vi "Display - Update_SubVI.vi"(4 "Error Msg In":string, 5 "Lat":dbl, 6 "Enum":T1, 7 "GPS Connected?":bool, 8 "error in (no error)":errorcluster, 9 "Heart Rate":dbl, 10 "Distance Run":dbl, 11 "Time Elapsed":dbl) -> (0 "error out":errorcluster)   [LabVIEW 2021]
uses:
  Main - States_SubVI.ctl
  <vilib>/myRIO/Instrument Drivers/Onboard IO/I2C/typedefs/I2C User Configuration.ctl
  <vilib>/myRIO/Instrument Drivers/Onboard IO/I2C/typedefs/I2C Transfer Rate.ctl
  <vilib>/myRIO/Instrument Drivers/Onboard IO/I2C/typedefs/I2C Reference.ctl
  <vilib>/myRIO/Common/Instrument Driver Framework/Utilities/typedefs/myRIO Generic Hardware Reference.ctl
  <vilib>/myRIO/Common/Instrument Driver Framework/Utilities/typedefs/Hardware Version Enum.ctl
  <vilib>/myRIO/Common/Instrument Driver Framework/Utilities/typedefs/myRIO v1.0 Reference.ctl
  <vilib>/myRIO/Common/Instrument Driver Framework/Utilities/typedefs/Generic FPGA Reference.ctl
  <vilib>/myRIO/Common/Instrument Driver Framework/myRIO v1.0/I2C/typedefs/I2C Channels Enum.ctl
  <vilib>/myRIO/Instrument Drivers/Onboard IO/I2C/typedefs/I2C Configuration.ctl
  <vilib>/userDefined/High Color/nirio_resource_hc.ctl
  <vilib>/myRIO/Common/Instrument Driver Framework/Utilities/vis/Is FPGA Ref Available.vi
  <vilib>/myRIO/Common/Instrument Driver Framework/myRIO v1.0/I2C/vis/myRIO v1.1 Open I2C.vi
  <vilib>/myRIO/Instrument Drivers/Onboard IO/I2C/vis/Configure.vi
  <vilib>/myRIO/Instrument Drivers/Onboard IO/I2C/vis/Write.vi
  <vilib>/myRIO/Common/Instrument Driver Framework/Utilities/vis/Validate Channels.vi
  <vilib>/myRIO/Common/Instrument Driver Framework/myRIO v1.0/I2C/vis/myRIO v1.0 Reserve I2C.vi
  <vilib>/myRIO/Common/Instrument Driver Framework/myRIO v1.0/I2C/vis/myRIO v1.0 Build MUX Configuration I2C.vi
  <vilib>/myRIO/Common/Instrument Driver Framework/myRIO v1.0/Resource Manager/vis/myRIO v1.0 Reserve Channel List.vi
  <vilib>/myRIO/Common/Instrument Driver Framework/myRIO v1.0/Resource Manager/vis/myRIO v1.0 Create Configuration List.vi
  <vilib>/myRIO/Common/Instrument Driver Framework/myRIO v1.0/Resource Manager/vis/myRIO v1.0 Reserve Channel.vi
  <vilib>/myRIO/Common/Instrument Driver Framework/myRIO v1.0/Resource Manager/vis/myRIO v1.0 Unreserve Channel.vi
  <vilib>/myRIO/Common/Instrument Driver Framework/myRIO v1.0/Resource Manager/vis/myRIO v1.0 Build Mutex Name.vi
  <vilib>/Utility/VariantDataType/GetNumericInfo.vi
  <vilib>/Utility/error.llb/Error Cluster From Error Code.vi
  <vilib>/myRIO/Common/Instrument Driver Framework/myRIO v1.0/myRIO v1.1 Open.vi
  <vilib>/myRIO/Common/Instrument Driver Framework/Utilities/vis/IO Manager.vi
  <vilib>/myRIO/Common/Instrument Driver Framework/Utilities/vis/Configuration Manager.vi
  <vilib>/myRIO/Common/Instrument Driver Framework/myRIO v1.0/Resource Manager/vis/myRIO v1.0 Configure IO.vi
  <vilib>/myRIO/Common/Instrument Driver Framework/myRIO v1.0/myRIO v1.0 Close.vi
  <vilib>/myRIO/Common/Instrument Driver Framework/myRIO v1.0/I2C/vis/myRIO v1.0 Configure I2C.vi
  <vilib>/myRIO/Common/Instrument Driver Framework/myRIO v1.0/I2C/vis/myRIO v1.0 Write I2C.vi
  <vilib>/myRIO/Express VI/Onboard IO/I2C/I2C Express VI.xnode
  <vilib>/myRIO/Instrument Drivers/Onboard IO/I2C/vis/myRIO I2C Open.xnode
  <vilib>/myRIO/Instrument Drivers/Onboard IO/I2C/I2C.lvlib
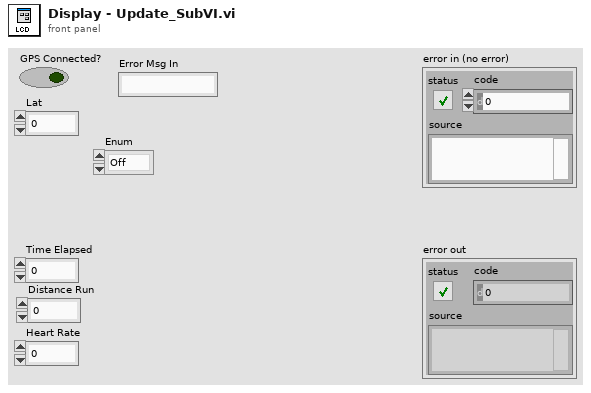
[diagram p1: front panel]
types:
  T1 = typedef "Main - States_SubVI.ctl" = enum16{"Off", "Record", "Upload", "Shutdown", "Error"}
  T2 = typedef "I2C.lvlib/I2C Reference.ctl" = cluster{"myRIO Reference":T3, "I2C Channels Enum":T7, "I2C Configuration":T8}
  T3 = typedef "myRIO Generic Hardware Reference.ctl" = cluster{"myRIO Model":T4, "myRIO Hardware Reference":T5}
  T4 = typedef "Hardware Version Enum.ctl" = enum16{"Unknown", "myRIO-1900", "myRIO-1950", "roboRIO", "NI ELVIS RIO CM", "ELVIS III"}
  T5 = typedef "myRIO v1.0 Reference.ctl" = cluster{"Generic FPGA Reference":T6, "Allow multiple opens":bool}
  T6 = typedef "Generic FPGA Reference.ctl" = refnum<k20>
  T7 = typedef "I2C Channels Enum.ctl" = enum16{"Not Connected", "A/I2C", "B/I2C", "I2C/I2C"}
  T8 = typedef "I2C.lvlib/I2C Configuration.ctl" = cluster{"I2C Transfer Rate":T9}
  T9 = typedef "I2C.lvlib/I2C Transfer Rate.ctl" = enum16{"Standard mode (100 kbps)", "Fast mode (400 kbps)"}
  T10 = typedef "I2C.lvlib/I2C User Configuration.ctl" = cluster{"I2C Transfer Rate":T9}
  T11 = typedef "nirio_resource_hc.ctl" = tag
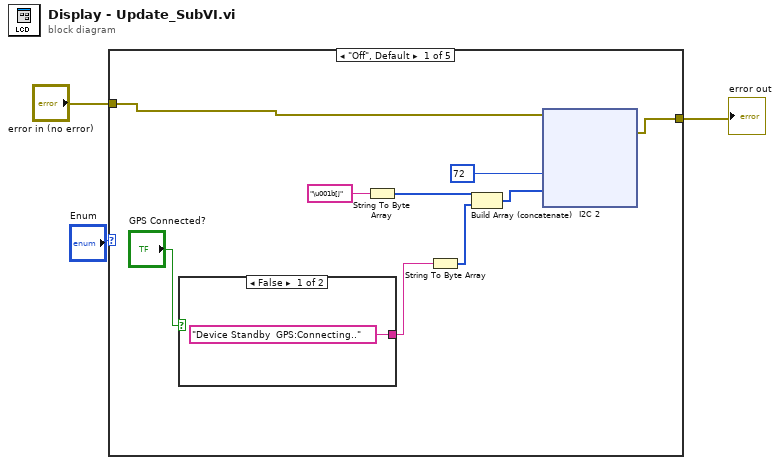
[diagram p0: block diagram]
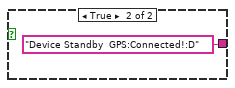
[diagram p2: hidden frame]
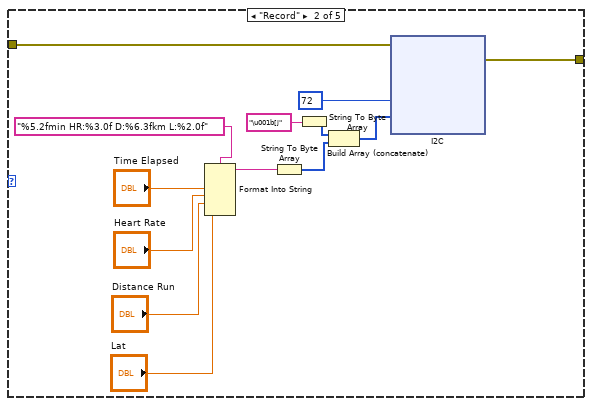
[diagram p3: hidden frame]
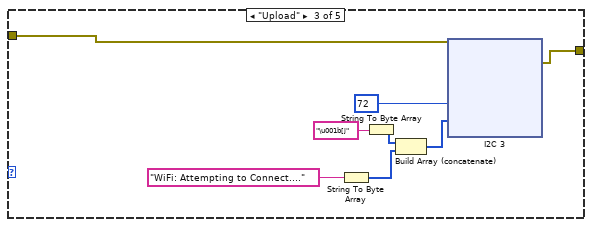
[diagram p4: hidden frame]
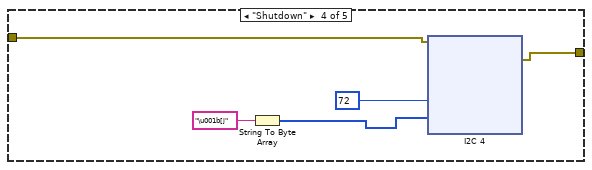
[diagram p5: hidden frame]
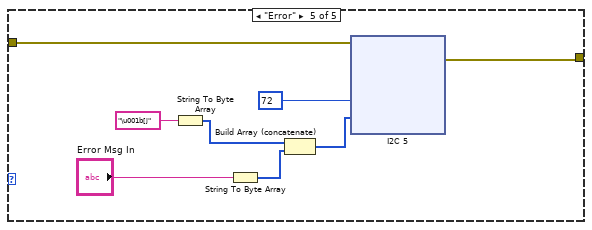
[diagram p6: hidden frame]
diagram:
  n1 = case shown="\"Off\", Default" "Enum" {
    tunnel: "error in (no error)" -> [w8 w61 w110 w152 w198]
    tunnel: [w11 w60 w109 w151 w197] -> w2
    frame "Off", Default {
      n2 = case shown="False" "GPS Connected?" {
        tunnel: ["Device Standby  GPS:Connecting.." ("format string") "Device Standby  GPS:Connected!:D" ("format string")] -> w9
        frame False {
        }
        frame True {
        }
      }
      n3 = String To Byte Array(string="\u001b[j") -> (unsigned byte array=w5:u8[])
      n4 = String To Byte Array(string=w9) -> (unsigned byte array=w7:u8[])
      n5 = Build Array (concatenate)(w5, w7) -> (w4:u8[])
      n6 = xnode "I2C 2"("Slave Address (7-bit)"=72, "Bytes to Write"=w4, "error in (no error)"=w8) -> ("error out"=w11:errorcluster)
    }
    frame "Record" {
      n7 = Format Into String(format string="%5.2fmin HR:%3.0f D:%6.3fkm L:%2.0f", "Time Elapsed", "Heart Rate", "Distance Run", "Lat") -> (resulting string=w59:string)  [unwired: 2 in, 1 out]
      n8 = String To Byte Array(string=w59) -> (unsigned byte array=w56:u8[])
      n9 = String To Byte Array(string="\u001b[j") -> (unsigned byte array=w57:u8[])
      n10 = Build Array (concatenate)(w57, w56) -> (w55:u8[])
      n11 = xnode "I2C"("Slave Address (7-bit)"=72, "Bytes to Write"=w55, "error in (no error)"=w61) -> ("error out"=w60:errorcluster)
    }
    frame "Upload" {
      n12 = String To Byte Array(string="WiFi: Attempting to Connect...." ("format string")) -> (unsigned byte array=w106:u8[])
      n13 = String To Byte Array(string="\u001b[j") -> (unsigned byte array=w107:u8[])
      n14 = Build Array (concatenate)(w107, w106) -> (w104:u8[])
      n15 = xnode "I2C 3"("Slave Address (7-bit)"=72, "Bytes to Write"=w104, "error in (no error)"=w110) -> ("error out"=w109:errorcluster)
    }
    frame "Shutdown" {
      n16 = String To Byte Array(string="\u001b[j") -> (unsigned byte array=w150:u8[])
      n17 = xnode "I2C 4"("Slave Address (7-bit)"=72, "Bytes to Write"=w150, "error in (no error)"=w152) -> ("error out"=w151:errorcluster)
    }
    frame "Error" {
      n18 = String To Byte Array(string="\u001b[j") -> (unsigned byte array=w195:u8[])
      n19 = String To Byte Array(string="Error Msg In") -> (unsigned byte array=w196:u8[])
      n20 = Build Array (concatenate)(w195, w196) -> (w194:u8[])
      n21 = xnode "I2C 5"("Slave Address (7-bit)"=72, "Bytes to Write"=w194, "error in (no error)"=w198) -> ("error out"=w197:errorcluster)
    }
  }
  "error out" <- w2
